vi "vi1.vi"() -> ()   [LabVIEW 2019]
panel:
  in  "x":i32
  out "x+y":i32
  in  "y":i32
  # "test"
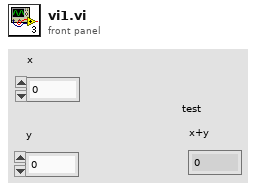
[diagram p1: front panel]
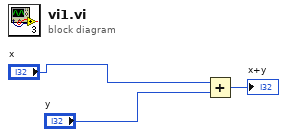
[diagram p0: block diagram]
diagram:
  n1 = Add(x="x", y="y") -> (x+y=→"x+y":i32)
